vi "integrate 1D array interval - double.vi"(2 "Ave N":dbl, 3 "Array In":dbl[](array[numeric])) -> (1 "Array Out":dbl[](array[numeric]))   [LabVIEW 2014]
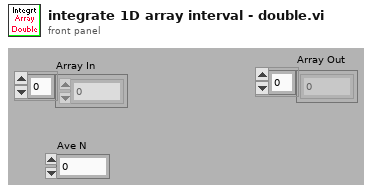
[diagram p1: front panel]
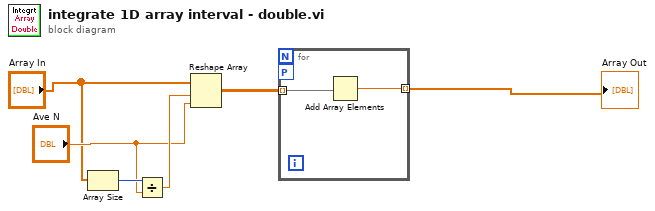
[diagram p0: block diagram]
diagram:
  n1 = Array Size(array="Array In") -> (size(s)=w6:i32)
  n2 = Divide(x=w6, y="Ave N") -> (x/y=w5:dbl)
  n3 = Reshape Array("Array In", w5, "Ave N") -> (w4:dbl[][])
  n4 = for {
    tunnel: w4 -> [w8] mode=indexing
    tunnel: [w7] -> w1 mode=indexing
    workers-P: _ -> [_]
    n5 = Add Array Elements(numeric array=w8) -> (sum=w7:dbl)
  }
  "Array Out" <- w1
